vi "Launcher.vi"   [LabVIEW 2025]
uses:
  Main/Main/Main.lvclass
  <vilib>/MGI/Panel Manager/Panel Actor/Panel Actor/Launch Root Panel Window.vi
  <vilib>/MGI/Panel Manager/Panel Actor/Panel Actor/Panel Actor.lvclass
panel:
  # "Loading, Please wait ...."
types:
  T1 = enum32{"Invalid", "Standard", "Closed", "Hidden", "Minimized", "Maximized"}
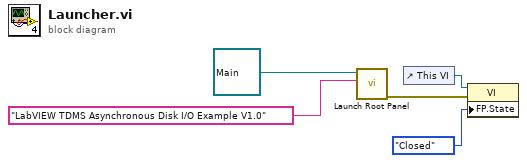
[diagram p0: block diagram]
diagram:
  n1 = call-poly <vilib>:"Launch Root Panel.vi"("Title"="LabVIEW TDMS Asynchronous Disk I/O Example V1.0", "Panel Actor in"=refnum<class "Main.lvclass"> refnum ("Main.lvlib:Main.lvclass")) -> ("Error Out"=w2:errorcluster)  [unwired: 8 in, 1 out]
  n2 = control-ref of="This VI"() -> (w3:refnum<vi>)
  n3 = property class="VI"(reference=w3, error in=w2, "FP.State"=T1."Closed" ("Front Panel Window:State")) -> ()  [unwired: 2 out]
